vi "NewSOC_req.vi"(6 "Static values":T3, 8 "error_in":errorcluster, 10 "Data Model":T4={"Time_control"=[], "P_ch_av (from grid)"=[], "PV_exc (W)"=[], "PV_exc (Wh)"=[], "Delta_t"=0.0, "Timestamp"=0, "SOC_end (array)"=[], "SOC_ini (array)"=[], "SOC_max_min"=[], "N_periods"=0, "SOC_end"=[], "SOC_ini"=[], "t_end"=[], "t_ini"=[], "Plugged"=[], "P_charge vs. SOC"={"SOC"=[0.0, 100.0], "P"=[3700.0, 3700.0]}, "SOC_ini_save"=[], "SOC_ini_save (array)"=[]}, 11 "Reqs_cluster":T2) -> (0 "error_out":errorcluster, 3 "SOC_reqs":T1)   [LabVIEW 2017]
uses:
  CONTROLS/Datamodel_FULL.ctl
  CONTROLS/P_ch_vs_SOC (array).ctl
  CONTROLS/Static_values.ctl
  CONTROLS/Reqs_cluster.ctl
  CONTROLS/SOC_reqs.ctl
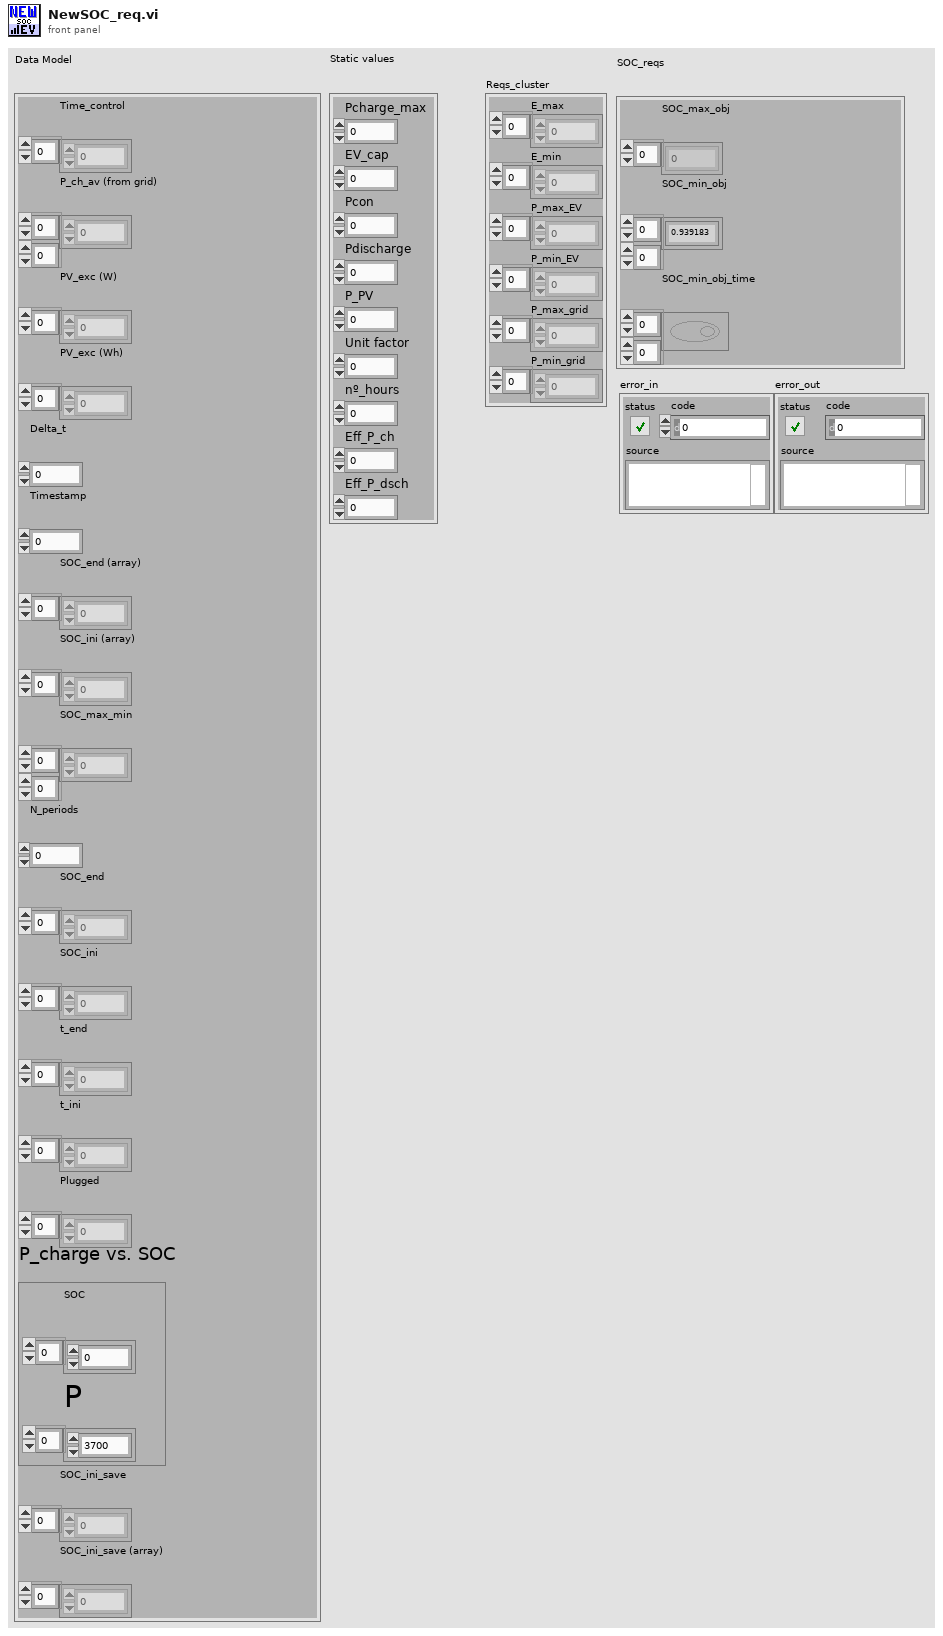
[diagram p1: front panel]
types:
  T1 = typedef "SOC_reqs.ctl" = cluster{"SOC_max_obj":dbl[], "SOC_min_obj":dbl[][], "SOC_min_obj_time":bool[][]}
  T2 = typedef "Reqs_cluster.ctl" = cluster{"E_max":dbl[], "E_min":dbl[], "P_max_EV":dbl[], "P_min_EV":dbl[], "P_max_grid":dbl[], "P_min_grid":dbl[]}
  T3 = typedef "Static_values.ctl" = cluster{"Pcharge_max":dbl, "EV_cap":dbl, "Pcon":dbl, "Pdischarge":dbl, "P_PV":dbl, "Unit factor":dbl, "nº_hours":dbl, "Eff_P_ch":dbl, "Eff_P_dsch":dbl}
  T4 = typedef "Datamodel_FULL.ctl" = cluster{"Time_control":i32[], "P_ch_av (from grid)":dbl[][], "PV_exc (W)":dbl[], "PV_exc (Wh)":dbl[], "Delta_t":dbl, "Timestamp":i32, "SOC_end (array)":dbl[], "SOC_ini (array)":dbl[], "SOC_max_min":dbl[][], "N_periods":i32, "SOC_end":dbl[], "SOC_ini":dbl[], "t_end":i32[], "t_ini":i32[], "Plugged":i32[], "P_charge vs. SOC":T5, "SOC_ini_save":dbl[], "SOC_ini_save (array)":dbl[]}
  T5 = typedef "P_ch_vs_SOC (array).ctl" = cluster{"SOC":dbl[], "P":dbl[]}
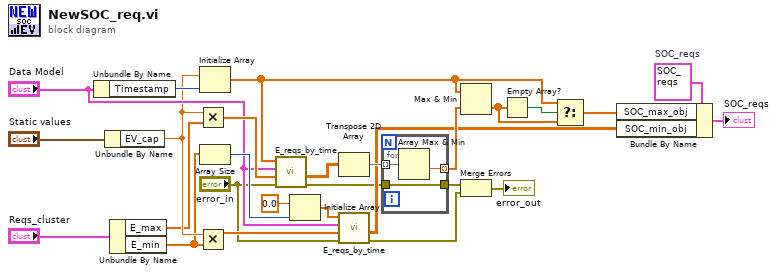
[diagram p0: block diagram]
diagram:
  w9 = T1 {"SOC_max_obj"=[], "SOC_min_obj"=array1x86400[86400 elements], "SOC_min_obj_time"=[]}  # SOC_reqs
  n1 = Unbundle By Name("Data Model") -> ("Timestamp"=w20:i32)
  n2 = Unbundle By Name("Static values") -> ("EV_cap"=w17:dbl)
  n3 = Unbundle By Name("Reqs_cluster") -> ("E_max"=w10:dbl[], "E_min"=w11:dbl[])
  n4 = Multiply(x=w17, y=w10) -> (x*y=w22:dbl[])
  n5 = Multiply(x=w17, y=w11) -> (x*y=w23:dbl[])
  n6 = Initialize Array(w17, w20) -> (w13:dbl[])
  n7 = Array Size(array=w11) -> (size(s)=w27:i32)
  n8 = call "E_reqs_by_time.vi"("error_in"="error_in", "E_req"=w22, "Data Model"="Data Model", "SOC_obj"=w13) -> ("error_out"=w3:errorcluster, "SOC_values"=w14:dbl[][])  [unwired: 4 in, 2 out]
  n9 = Initialize Array(0.0 ("element"), w27) -> (w15:dbl[])
  n10 = Transpose 2D Array(2D array=w14) -> (transposed array=w26:dbl[][])
  n11 = call "E_reqs_by_time.vi"("error_in"="error_in", "E_req"=w23, "Data Model"="Data Model", "SOC_obj"=w15) -> ("error_out"=w4:errorcluster, "SOC_values"=w7:dbl[][])  [unwired: 4 in, 2 out]
  n12 = for {
    tunnel: w26 -> [w30] mode=indexing
    tunnel: [w29] -> w25 mode=indexing
    tunnel: [w28] -> w2
    tunnel: w3 -> [w28]
    n13 = Array Max & Min(array=w30) -> (min value=w29:dbl)  [unwired: 3 out]
  }
  n14 = Max & Min(x=w13, y=w25) -> (min(x,y)=w18:dbl[])  [unwired: 1 out]
  n15 = Merge Errors(w2, w4) -> (→"error_out":errorcluster)
  n16 = Empty Array?(array=w18) -> (empty?=w19:bool)
  n17 = Select(t=w13, s=w19, f=w18) -> (s? t:f=w8:dbl[])
  n18 = Bundle By Name(cluster=w9, "SOC_max_obj"=w8, "SOC_min_obj"=w7) -> (→"SOC_reqs":T1)
